vi "Get Supported Targets.vi"(8 "error in":errorcluster, 11 "Standard Engine Repo Data in":refnum<class "synchronous engine configuration.lvclass">) -> (0 "error out":errorcluster, 2 "Supported Targets":T1[](array[typedef]), 3 "Standard Engine Repo Data out":refnum<class "synchronous engine configuration.lvclass">)   [LabVIEW 2013, in "synchronous engine configuration.lvclass"]
uses:
  synchronous engine configuration.lvclass
  <vilib>/NI/Tag Bus Module Framework/root configuration/Target Types.ctl
  <vilib>/NI/Tag Bus Module Framework/root configuration/TBM configuration.lvclass
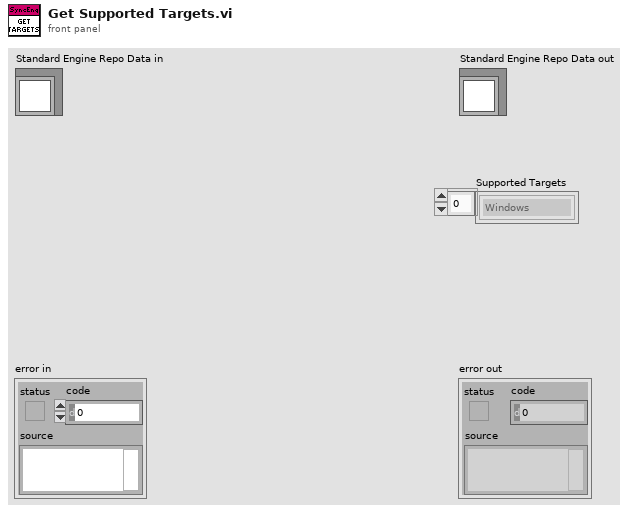
[diagram p1: front panel]
types:
  T1 = typedef "TBM configuration.lvclass/Target Types.ctl" = enum16{"Windows", "Mac", "Linux", "Linux RT ARM", "VxWorks", "Pharlap", "Other", "Linux RT x64"}
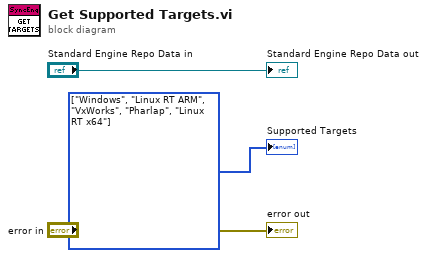
[diagram p0: block diagram]
diagram:
  w1 = T1[] [enum."Windows", enum."Linux RT ARM", enum."VxWorks", enum."Pharlap", enum."Linux RT x64"] items=["Windows", "Mac", "Linux", "Linux RT ARM", "VxWorks", "Pharlap", "Other", "Linux RT x64"] ("Supported Targets")
  "error out" <- "error in"
  "Standard Engine Repo Data out" <- "Standard Engine Repo Data in"
  "Supported Targets" <- w1
